vi "Initialize.vi"(7 "Serial Configuration":T1={"Baud Rate"=115200, "Parity"=0, "Data Bits"=8, "Stop Bits"=10, "Flow Control"=0} {"Flow Control" items=["None", "XON/XOFF", "RTS/CTS", "XON/XOFF & RTS/CTS", "DTR/DSR", "XON/XOFF & DTR/DSR"]; "Stop Bits" items=["1.0"=10, "1.5"=15, "2.0"=20]; "Data Bits" items=["7"=7, "8"=8]; "Parity" items=["None", "Odd", "Even", "Mark", "Space"]; "Baud Rate" items=["300"=300, "600"=600, "1200"=1200, "2400"=2400, "4800"=4800, "9600"=9600, "19200"=19200]}, 8 "error in (no error)":errorcluster, 10 "ID Query (True)":bool=TRUE, 11 "VISA resource name":refnum<visa-resource-name>="COM8") -> (0 "error out":errorcluster, 2 "ID String":string, 3 "VISA resource name out":refnum<visa-resource-name>)   [LabVIEW 2025, in "Detector SCPI.lvlib"]
doc: "Establishes communication with the instrument and optionally performs an instrument identification query and/or an instrument reset. It also places the instrument in a default state needed for other instrument driver operations. Therefore, call this VI before calling other instrument driver VIs for this instrument. Generally, you need to call the <b>Initialize</b> VI only once at the beginning of an application."
uses:
  Detector SCPI.lvlib
panel:
  # "(c) 2014 <Enter Company Name Here>.  ALL RIGHTS RESERVED."
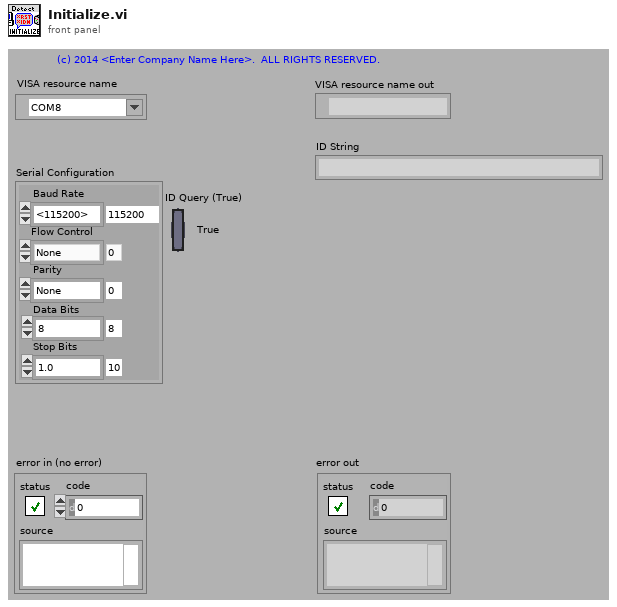
[diagram p1: front panel]
types:
  T1 = cluster{"Baud Rate":u32, "Parity":u16, "Data Bits":u16, "Stop Bits":u16, "Flow Control":u16}
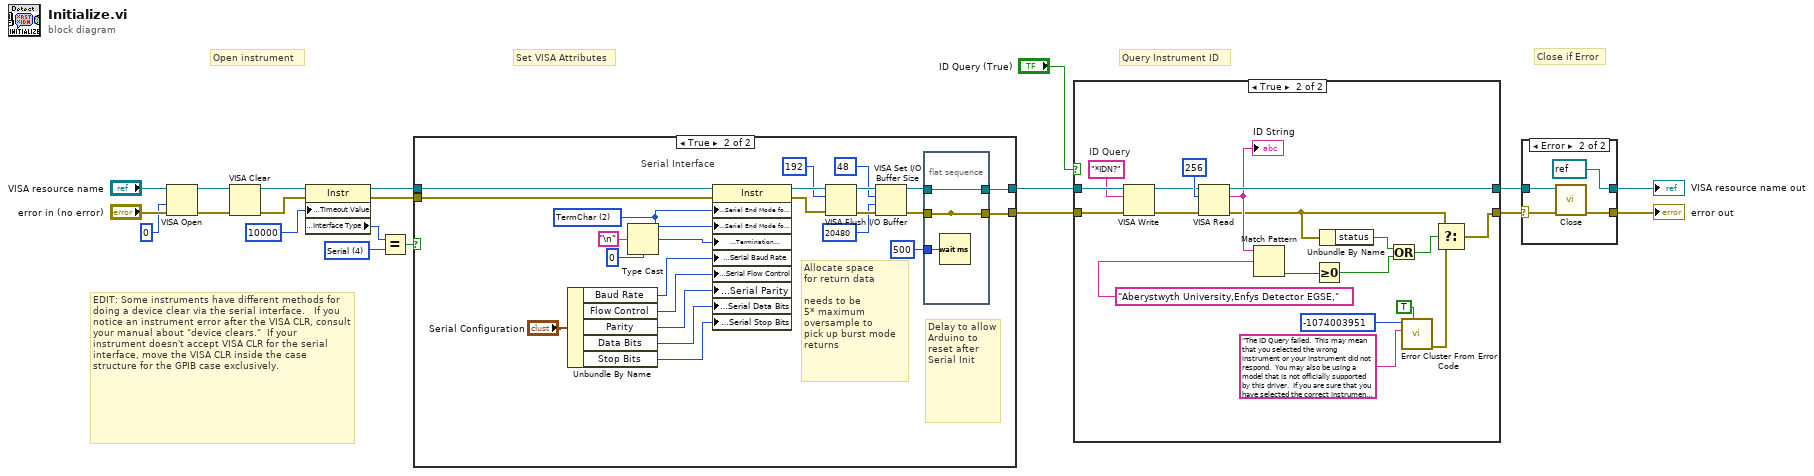
[diagram p0: block diagram]
diagram:
  w8 = u16 4 items=["GPIB"=1, "VXI"=2, "GPIB-VXI"=3, "Serial"=4, "PXI"=5, "TCPIP"=6, "USB"=7] ("Interface Information:Interface Type")
  # "EDIT: Some instruments have different methods for doing a device clear via the serial interface.   If you notice an instrument error after the VISA CLR, consult your manual about \"device clears.\"  If your instrument doesn't accept VISA CLR for the serial interface, move the VISA CLR inside the case  structure for the GPIB case exclusively."
  # "Set VISA Attributes"
  # "Close if Error"
  # "Query Instrument ID"
  # "Open instrument"
  n1 = VISA Open(access mode=u32 0, error in (no error)="error in (no error)", VISA resource name="VISA resource name") -> (VISA resource name=w6:refnum<visa-resource-name>, error out=w5:errorcluster)  [unwired: 2 in]
  n2 = VISA Clear(VISA resource name=w6, error in (no error)=w5) -> (VISA resource name out=w4:refnum<visa-resource-name>, error out=w3:errorcluster)
  n3 = property class="Instr"(reference=w4, error in=w3, "General Settings:Timeout Value"=u32 10000) -> (reference out=w11:refnum<visa-resource-name>, error out=w10:errorcluster, "Interface Information:Interface Type"=w15:u16)
  n4 = Equal?(x=w15, y=w8) -> (x = y?=w9:bool)
  n5 = case shown="True" w9 {
    tunnel: [w21 w26] -> w13
    tunnel: [w22 w24] -> w12
    tunnel: w11 -> [w21 w45]
    tunnel: w10 -> [w22 w46]
    frame False {
      # "EDIT: Remove interfaces not supported by your instrument."
      # "GPIB, TCP/IP, and USB Interface"
    }
    frame True {
      w35 = u16 2 items=["None", "LastBit", "TermChar"] ("Serial Settings:Serial End Mode for Reads")
      # "Allocate space \nfor return data\n\nneeds to be \n5* maximum\noversample to\npick up burst mode\nreturns"
      # "Delay to allow \nArduino to reset after\nSerial Init"
      # "Serial Interface"
      n6 = Unbundle By Name("Serial Configuration") -> ("Baud Rate"=w33:u32, "Flow Control"=w29:u16, "Parity"=w31:u16, "Data Bits"=w32:u16, "Stop Bits"=w28:u16)
      n7 = Type Cast(type=u8 0, x="\n") -> (*(type *) &x=w34:u8)
      n8 = property class="Instr"(reference=w45, error in=w46, "Serial Settings:Serial End Mode for Reads"=w35, "Serial Settings:Serial End Mode for Writes"=w35, "Message Based Settings:Termination Character"=w34, "Serial Settings:Serial Baud Rate"=w33, "Serial Settings:Serial Flow Control"=w29, "Serial Settings:Serial Parity"=w31, "Serial Settings:Serial Data Bits"=w32, "Serial Settings:Serial Stop Bits"=w28) -> (reference out=w41:refnum<visa-resource-name>, error out=w43:errorcluster)
      n9 = VISA Flush I/O Buffer(VISA resource name=w41, mask (16)=u16 192, error in (no error)=w43) -> (VISA resource name out=w44:refnum<visa-resource-name>, error out=w42:errorcluster)
      n10 = VISA Set I/O Buffer Size(VISA resource name=w44, mask (16)=u16 48, size (4096)=u32 20480 ("size (0)"), error in (no error)=w42) -> (VISA resource name out=w27:refnum<visa-resource-name>, error out=w25:errorcluster)
      n11 = flat-sequence {
        tunnel: w27 -> [w49]
        tunnel: [w49] -> w26
        tunnel: 500 ("Delay(ms)") -> [w48]
        tunnel: w25 -> [w47]
        tunnel: [w47] -> _
        tunnel: [w47] -> w24
        frame #0 {
          n12 = Wait (ms)(milliseconds to wait=w48) -> ()  [unwired: 1 out]
        }
      }
    }
  }
  n13 = case shown="True" "ID Query (True)" {
    tunnel: [w50 w70] -> w19
    tunnel: [w51 w67] -> w20
    tunnel: w13 -> [w51 w68]
    tunnel: w12 -> [w50 w69]
    frame False {
    }
    frame True {
      w65 = "*IDN?"  # ID Query
      n14 = VISA Write(VISA resource name=w68, write buffer=w65, error in (no error)=w69) -> (VISA resource name out=w54:refnum<visa-resource-name>, error out=w53:errorcluster)  [unwired: 1 out]
      n15 = VISA Read(VISA resource name=w54, byte count=u32 256 ("Bytes at Port"), error in (no error)=w53) -> (VISA resource name out=w67:refnum<visa-resource-name>, read buffer=w66:string, error out=w59:errorcluster)  [unwired: 1 out]
      "ID String" <- w66
      n16 = Match Pattern(string=w66, regular expression="Aberystwyth University,Enfys Detector EGSE,") -> (offset past match=w60:i32)  [unwired: 1 in, 3 out]
      n17 = Greater Or Equal To 0?(x=w60) -> (x >= 0?=w57:bool)
      n18 = Unbundle By Name(w59) -> ("status"=w58:bool)
      n19 = Or(x=w58, y=w57) -> (x .or. y?=w56:bool)
      n20 = call <vilib>:"Error Cluster From Error Code.vi"("show call chain? (False)"=TRUE, "error message (\"\")"="The ID Query failed.  This may mean that you selected the wrong instrument or your instrument did not respond.  You may also be using a model that is not officially supported by this driver.  If you are sure that you have selected the correct instrument and it is responding, try disabling the ID Query." ("Source (VI Name)"), "error code (0)"=-1074003951 ("Code")) -> ("error out"=w64:errorcluster)  [unwired: 6 in]
      n21 = Select(t=w59, s=w56, f=w64) -> (s? t:f=w70:errorcluster)
    }
  }
  n22 = case shown="Error" w19 {
    selector: w19 -> [w71 w74]
    tunnel: w20 -> [w72 w75]
    tunnel: [w72 refnum<visa-resource-name> refnum ("VISA resource name out")] -> w2
    tunnel: [w71 w76] -> w1
    frame No Error {
    }
    frame Error {
      n23 = call "Close.vi"("error in (no error)"=w74, "VISA resource name"=w75) -> ("error out"=w76:errorcluster)  [unwired: 9 in]
    }
  }
  "VISA resource name out" <- w2
  "error out" <- w1
